vi "RPC Test Library Path.vi"(9 "Test ID (\"\")":string, 10 "Base Path (empty)":path, 11 "App Ref (null: local)":refnum<vi>) -> (1 "Component Name":string, 2 "Library Path":path, 3 "dup App Ref":refnum<vi>)   [LabVIEW 2011]
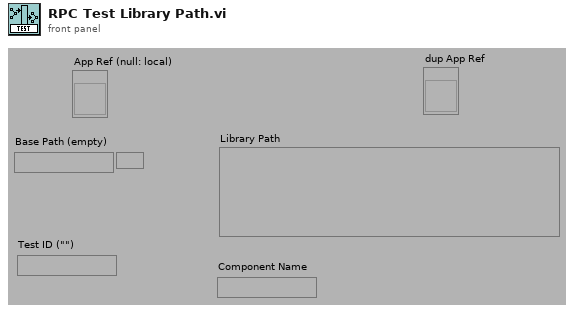
[diagram p1: front panel]
types:
  T1 = enum32{"invalid app kind", "Development System", "Run Time System", "Student Edition", "Embedded LabVIEW", "Evaluation", "Custom"}
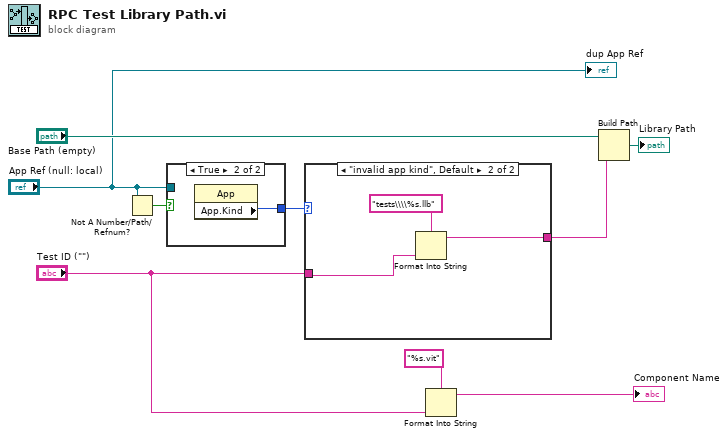
[diagram p0: block diagram]
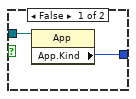
[diagram p2: hidden frame]
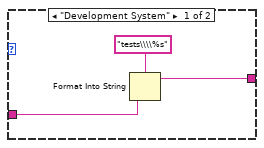
[diagram p3: hidden frame]
diagram:
  n1 = Not A Number/Path/Refnum?(number/path/refnum="App Ref (null: local)") -> (NaN/Path/Refnum?=w3:bool)
  n2 = case shown="True" w3 {
    tunnel: [w11 w12] -> w2
    tunnel: "App Ref (null: local)" -> [w10 _]
    frame False {
      n3 = property class="App"(reference=w10) -> ("App.Kind"=w11:T1)  [unwired: 1 in, 2 out]
    }
    frame True {
      n4 = property class="App"() -> ("App.Kind"=w12:T1)  [unwired: 2 in, 2 out]
    }
  }
  n5 = case shown="\"invalid app kind\", Default" w2 {
    tunnel: [w14 w17] -> w9
    tunnel: "Test ID (\"\")" -> [w13 w16]
    frame "Development System" {
      n6 = Format Into String(format string="tests\\\\%s", w13) -> (resulting string=w14:string)  [unwired: 2 in, 1 out]
    }
    frame "invalid app kind", Default {
      n7 = Format Into String(format string="tests\\\\%s.llb", w16) -> (resulting string=w17:string)  [unwired: 2 in, 1 out]
    }
  }
  n8 = Format Into String(format string="%s.vit", "Test ID (\"\")") -> (resulting string=→"Component Name":string)  [unwired: 2 in, 1 out]
  n9 = Build Path(base path="Base Path (empty)", name or relative path=w9) -> (appended path=→"Library Path":path)
  "dup App Ref" <- "App Ref (null: local)"
